vi "PK FGV.vi"(10 "Enum":T1, 11 "Array":string[](array[string])) -> (3 "Array 2":string[](array[string]))   [LabVIEW 2015, in "Copy of Untitled Library 1.lvlib"]
uses:
  Copy of Untitled Library 1.lvlib
  Controls/Control FGVPK.ctl
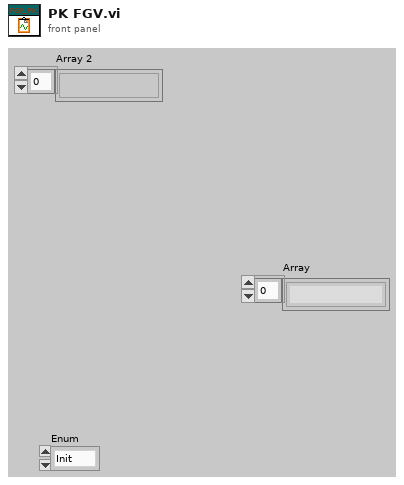
[diagram p1: front panel]
types:
  T1 = typedef "Control FGVPK.ctl" = enum16{"Init", "Read", "write", ""}
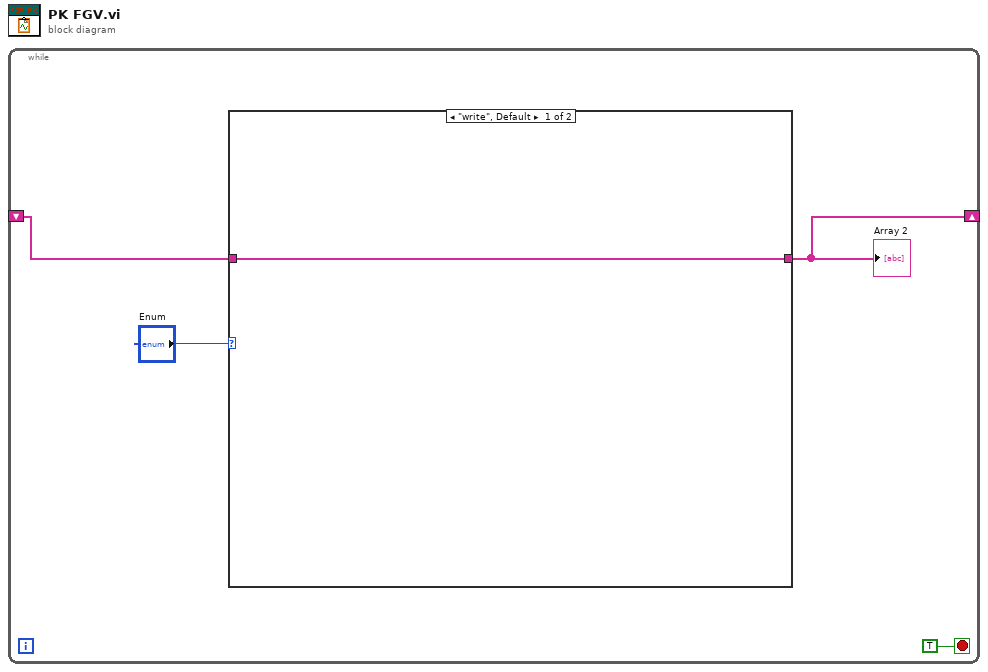
[diagram p0: block diagram]
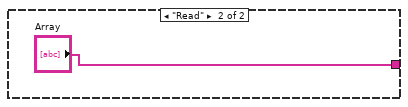
[diagram p2: hidden frame]
diagram:
  n1 = while {
    shift-right: [w2] -> _
    shift-left: _ -> [w1]
    stop <- TRUE stop-if-true
    n2 = case shown="\"write\", Default" "Enum" {
      tunnel: [w5 "Array"] -> w2
      tunnel: w1 -> [w5 _]
      frame "write", Default {
      }
      frame "Read" {
      }
    }
    "Array 2" <- w2
  }
